vi "AutoDrive_sub.vi"(8 "EncoderVals":i32[](array[numeric]), 9 "Target Heading (Degrees)":i16, 10 "Drive Control":T2={"Left X"=0, "Left Y"=0, "Right X"=0, "Power (100)"=100, "Wait (ms)"=100, "Enc/Deg Target"=0, "Move Type"=enum."Wait"} {"Power (100)" min=-100 max=100}, 11 "NXT/EV3":T1) -> (0 "EncoderVals":i32[](array[numeric]), 3 "NXT/EV3 out":T1)   [LabVIEW 2012, in "Mecanum Drive.lvrbt"]
uses:
  Mecanum Drive.lvrbt
  <vilib>/NXT/Hardware/Plugins/Tetrix DC Motor/TetrixDCMotorAddress.ctl
  <vilib>/NXT/LegoClasses/BrickReference/BrickReference.lvclass
  <vilib>/NXT/Subs/LVHSConnector.ctl
  <vilib>/NXT/NXTIO Xnodes/NXTIONodeSubVIs/TETRIX IO Move DC Motors.vi
  <vilib>/NXT/NXTIO Xnodes/NXTIOXNode/NXTIO.xnode
  <vilib>/NXT/NXTIO Xnodes/AddressXNode/NXTIOAddress.xnode
  <vilib>/FTC/FTC POVState.ctl
  <vilib>/FTC/FTC ControllerState.ctl
  <vilib>/NXT/NXTIO Xnodes/NXTIONodeSubVIs/TETRIX IO Motor Status.vi
  <vilib>/NXT/Block Support/NXT_InputPort.ctl
  <vilib>/NXT/HiTechnic/HiTechnic Controls/HiTechnic Port.ctl
  <vilib>/NXT/Dual Mode Library/Waits/Wait_Num(msec).vi
  <vilib>/NXT/Dual Mode Library/Display/drawNumber.vi
  SubVIs/auto_drive_TYP.ctl
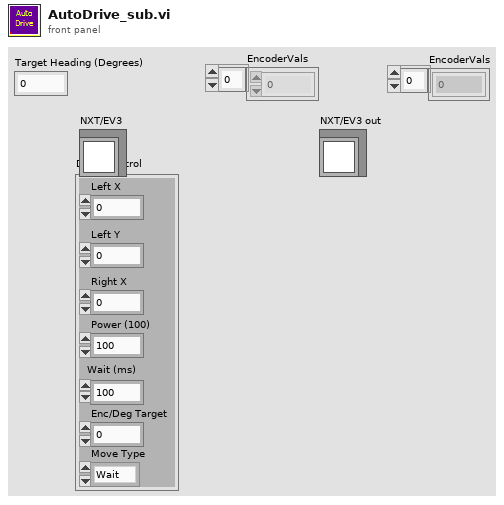
[diagram p1: front panel]
types:
  T1 = typedef "LVHSConnector.ctl" = refnum<class "BrickReference.lvclass">
  T2 = typedef "auto_drive_TYP.ctl" = cluster{"Left X":i8, "Left Y":i8, "Right X":i8, "Power (100)":i8, "Wait (ms)":u32, "Enc/Deg Target":i32, "Move Type":enum16{"Relative Degrees", "Wait", "Encoder"}}
  T3 = typedef "FTC ControllerState.ctl" = cluster{"Left X":i8, "Left Y":i8, "Right X":i8, "Right Y":i8, "Button Encoding 9-12":u8, "Button Encoding 1-8":u8, "POV":T4}
  T4 = typedef "FTC POVState.ctl" = i8
  T5 = typedef "TetrixDCMotorAddress.ctl" = i32
  T6 = typedef "HiTechnic Port.ctl" = cluster{"Port":T7, "MUX Port":u8}
  T7 = typedef "NXT_InputPort.ctl" = u32
  T8 = cluster{"TetrixDCMotor":T5, "TetrixDCMotor 2":T5}
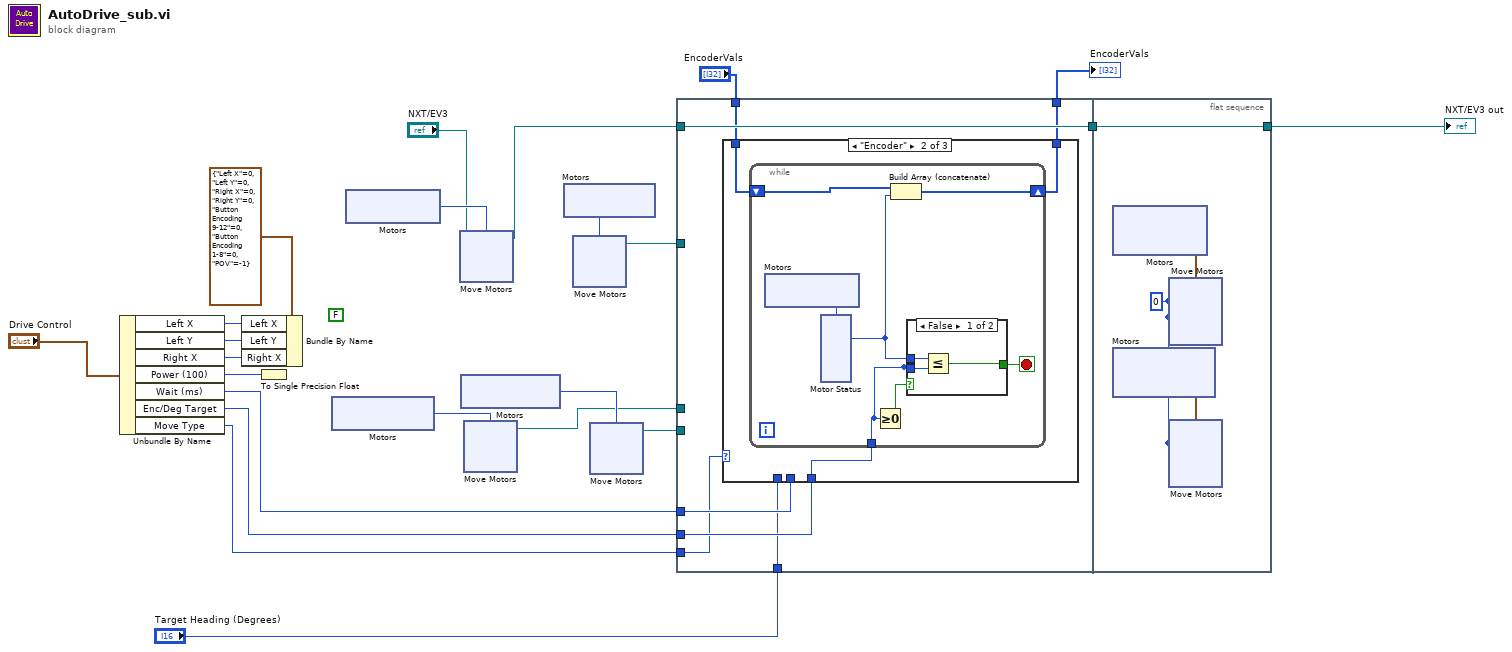
[diagram p0: block diagram]
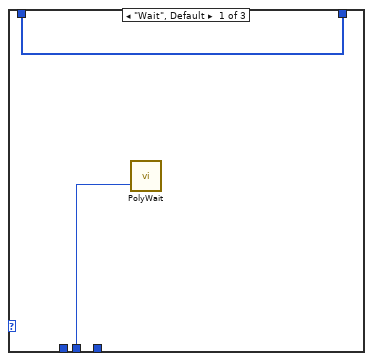
[diagram p2: hidden frame]
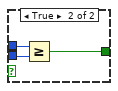
[diagram p3: hidden frame]
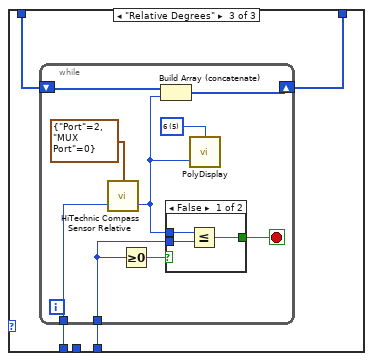
[diagram p4: hidden frame]
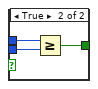
[diagram p5: hidden frame]
diagram:
  (unwired) FALSE
  n1 = Unbundle By Name("Drive Control") -> ("Left X"=w17:i8, "Left Y"=w16:i8, "Right X"=w15:i8, "Power (100)"=w9:i8, "Wait (ms)"=w10:u32, "Enc/Deg Target"=w5:i32, "Move Type"=w4:enum16{"Relative Degrees", "Wait", "Encoder"})
  n2 = Bundle By Name(cluster=T3 {"Left X"=0, "Left Y"=0, "Right X"=0, "Right Y"=0, "Button Encoding 9-12"=0, "Button Encoding 1-8"=0, "POV"=-1} ("Controller State"), "Left X"=w17, "Left Y"=w16, "Right X"=w15) -> ()  [unwired: 1 out]
  n3 = To Single Precision Float(number=w9) -> (single precision float=w8:sgl)
  n4 = xnode ("Motors")() -> ("Motor"=w28:T5)
  n5 = xnode ("Motors")() -> ("Motor"=w25:T5)
  n6 = xnode ("Move Motors")("Motors"=w25, "NXT/EV3"="NXT/EV3") -> ("Power/Speed 1"=w21:i8, "NXT/EV3"=w14:T1)
  n7 = xnode ("Motors")() -> ("Motor"=w27:T5)
  n8 = xnode ("Move Motors")("Motors"=w28) -> ("Power/Speed 1"=w23:i8, "NXT/EV3"=w11:T1)  [unwired: 1 in]
  n9 = xnode ("Motors")() -> ("Motor"=w26:T5)
  n10 = xnode ("Move Motors")("Motors"=w26) -> ("Power/Speed 1"=w24:i8, "NXT/EV3"=w13:T1)  [unwired: 1 in]
  n11 = xnode ("Move Motors")("Motors"=w27) -> ("Power/Speed 1"=w22:i8, "NXT/EV3"=w12:T1)  [unwired: 1 in]
  n12 = flat-sequence {
    tunnel: w14 -> [w35]
    tunnel: w13 -> [_]
    tunnel: w12 -> [_]
    tunnel: w11 -> [_]
    tunnel: w10 -> [w34]
    tunnel: [w35] -> w6
    tunnel: w5 -> [w33]
    tunnel: w4 -> [w32]
    tunnel: "Target Heading (Degrees)" -> [w31]
    tunnel: "EncoderVals" -> [w30]
    tunnel: [w29] -> w1
    tunnel: [w85] -> w7
    tunnel: w6 -> [w85]
    frame #0 {
      n13 = case shown="\"Encoder\"" w32 {
        tunnel: w34 -> [w37 _ _]
        tunnel: w33 -> [_ w40 w65]
        tunnel: w31 -> [_ _ w66]
        tunnel: w30 -> [w36 w39 w64]
        tunnel: [w36 w38 w63] -> w29
        frame "Wait", Default {
          n14 = call-poly <vilib>:"PolyWait.vi"("Time (100 msec)"=w37) -> ()  [unwired: 3 in, 1 out]
        }
        frame "Encoder" {
          n15 = while {
            tunnel: w40 -> [w41]
            shift-right: [w46] -> w38
            shift-left: w39 -> [w45]
            stop <- w42 stop-if-true
            n16 = xnode "Motors"() -> ("Motor"=w47:T5)
            n17 = xnode "Motor Status"("Motors"=w47) -> ("Position 1"=w43:i32)  [unwired: 1 in, 2 out]
            n18 = Greater Or Equal To 0?(x=w41) -> (x >= 0?=w44:bool)
            n19 = Build Array (concatenate)(w45, w43) -> (w46:i32[])
            n20 = case shown="False" w44 {
              tunnel: w41 -> [_ w52]
              tunnel: w43 -> [w50 w53]
              tunnel: [w48 w51] -> w42
              tunnel: w41 -> [w49 _]
              frame False {
                n21 = Less Or Equal?(x=w50, y=w49) -> (x <= y?=w48:bool)
              }
              frame True {
                n22 = Greater Or Equal?(x=w53, y=w52) -> (x >= y?=w51:bool)
              }
            }
          }
        }
        frame "Relative Degrees" {
          n23 = while {
            tunnel: w66 -> [w74]
            tunnel: w65 -> [w71]
            shift-right: [w69] -> w63
            shift-left: w64 -> [w67]
            stop <- w73 stop-if-true
            w72 = i16 5 items=["1", "2", "3", "4", "5", "6", "7", "8", "9", "10", "11", "12"] ("Line")
            n24 = call <vilib>:"HiTechnic Compass Sensor Relative.vi"("Target Heading (Degrees)"=w74, "Port/MUX"=T6 {"Port"=2, "MUX Port"=0}) -> ("Relative Heading (Degrees)"=w68:i32)  [unwired: 1 in, 1 out]
            n25 = Greater Or Equal To 0?(x=w71) -> (x >= 0?=w70:bool)
            n26 = Build Array (concatenate)(w67, w68) -> (w69:i32[])
            n27 = case shown="False" w70 {
              tunnel: w71 -> [w76 w81]
              tunnel: [w78 w80] -> w73
              tunnel: w68 -> [w77 w79]
              frame False {
                n28 = Less Or Equal?(x=w77, y=w76) -> (x <= y?=w78:bool)
              }
              frame True {
                n29 = Greater Or Equal?(x=w79, y=w81) -> (x >= y?=w80:bool)
              }
            }
            n30 = call-poly <vilib>:"PolyDisplay.vi"("number"=w68, "Line"=w72) -> ()  [unwired: 2 in, 1 out]
          }
        }
      }
    }
    frame #1 {
      w82 = i8 0 ("Power/Speed 1")
      n31 = xnode "Motors"() -> ("Motor"=w84:cluster{"TetrixDCMotor":T5, "TetrixDCMotor":T5})
      n32 = xnode "Motors"() -> ("Motor"=w83:cluster{"TetrixDCMotor":T5, "TetrixDCMotor":T5})
      n33 = xnode "Move Motors"("Power/Speed 2"=w82, "Power/Speed 1"=w82, "Motors"=w84) -> ()  [unwired: 1 in, 1 out]
      n34 = xnode "Move Motors"("Power/Speed 2"=w82, "Power/Speed 1"=w82, "Motors"=w83) -> ()  [unwired: 1 in, 1 out]
    }
  }
  "NXT/EV3 out" <- w7
  "EncoderVals" <- w1
